vi "open documentation by name.vi"(8 "error in (no error)":errorcluster, 10 "base class":string, 11 "path to XML documents":path) -> (0 "error out":errorcluster, 3 "Refnum out":refnum<k20>)   [LabVIEW 2023]
uses:
  <vilib>/xml/Load XML File.vi
  <vilib>/xml/NI_XML.lvlib
panel:
  out "parse errors":string
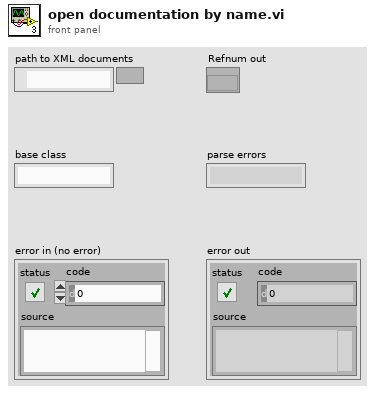
[diagram p1: front panel]
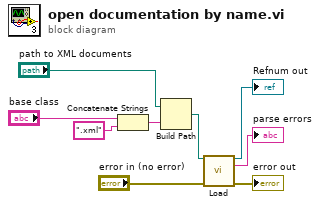
[diagram p0: block diagram]
diagram:
  n1 = Concatenate Strings("base class", ".xml" ("string")) -> (w7:string)
  n2 = Build Path(base path="path to XML documents", name or relative path=w7) -> (appended path=w8:path)
  n3 = call-poly <vilib>:"Load.vi"("path to XML document"=w8, "error in (no error)"="error in (no error)") -> ("DOM document out"=→"Refnum out":refnum<k20>, "parse errors"=→"parse errors":string, "error out"=→"error out":errorcluster)  [unwired: 11 in]
